vi "System Exec.vi"(8 "error in (no error)":errorcluster, 10 "standard input":string, 11 "subprocess in":refnum<class "Subprocess.lvclass">) -> (0 "error out":errorcluster, 1 "standard error":string, 2 "standard output":string, 3 "subprocess out":refnum<class "Subprocess.lvclass">, 4 "return code":i32)   [LabVIEW 2020, in "NI_Subprocess.lvlib" / "Subprocess.lvclass"]
doc: "Execute the configured command with System Exec."
uses:
  <vilib>/Subprocess/Subprocess/Subprocess.lvclass
  <vilib>/Subprocess/Subprocess/Subprocess.lvclass/Subprocess.ctl
  <vilib>/Utility/error.llb/Error Cluster From Error Code.vi
  <vilib>/ErrorRing/Error Ring.xnode
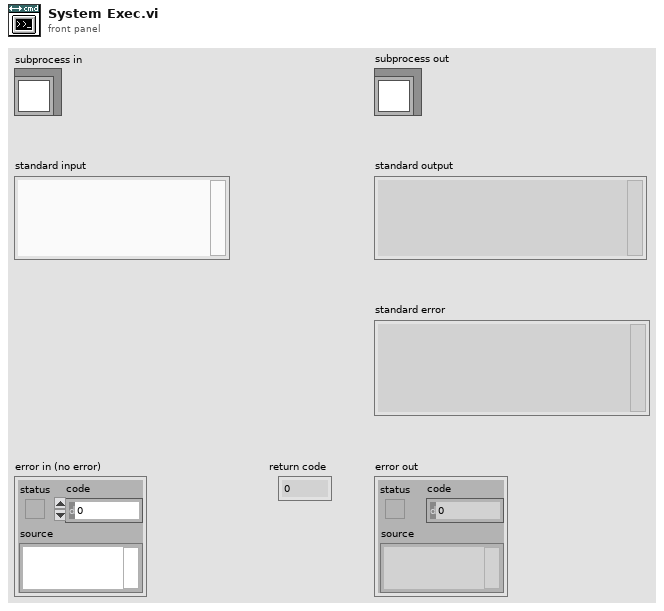
[diagram p1: front panel]
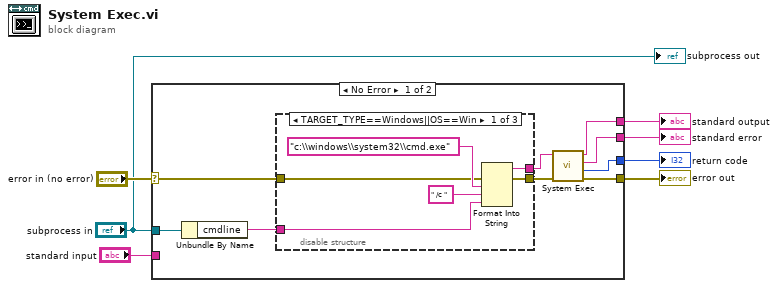
[diagram p0: block diagram]
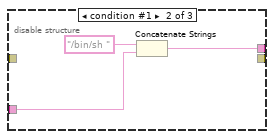
[diagram p2: hidden frame]
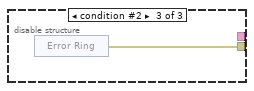
[diagram p3: hidden frame]
diagram:
  n1 = case shown="No Error" "error in (no error)" {
    selector: "error in (no error)" -> [w16 w31]
    tunnel: [w12 w31] -> w6
    tunnel: "subprocess in" -> [w15 _]
    tunnel: "standard input" -> [_ _]
    tunnel: [w9 _] -> w4
    tunnel: [w8 _] -> w3
    tunnel: [w10 _] -> w2
    frame No Error {
      n2 = Unbundle By Name(w15) -> ("cmdline"=w14:string)
      n3 = disable-structure shown="TARGET_TYPE==Windows||OS==Win" {
        disable-tunnel: w16 -> [w20 _ _]
        disable-tunnel: [w18 _ w26] -> w13
        disable-tunnel: w14 -> [w19 w24 _]
        disable-tunnel: [w17 w23 _] -> w11
        frame condition #0 (active) {
          n4 = Format Into String(error in=w20, "c:\\windows\\system32\\cmd.exe", " /c " ("input 2"), w19) -> (resulting string=w17:string, error out=w18:errorcluster)  [unwired: 2 in]
        }
        frame condition #1 {
          n5 = Concatenate Strings("/bin/sh ", w24) -> (w23:string)
        }
        frame condition #2 {
          n6 = xnode "Error Ring"() -> ("error out"=w26:errorcluster)
        }
      }
      n7 = call <vilib>:"System Exec.vi"("error in (no error)"=w13, "command line"=w11) -> ("error out"=w12:errorcluster, "return code"=w10:i32, "standard error"=w8:string, "standard output"=w9:string)  [unwired: 6 in]
    }
    frame Error {
    }
  }
  "error out" <- w6
  "standard output" <- w4
  "standard error" <- w3
  "return code" <- w2
  "subprocess out" <- "subprocess in"
